vi "DestroyPublicEvents.vi"(8 "error in (no error)":errorcluster, 11 "JKI.Robot.SMO":refnum<class "JKI.Robot.SMO.lvclass">) -> (0 "error out":errorcluster, 3 "JKI.Robot.SMO out":refnum<class "JKI.Robot.SMO.lvclass">)   [LabVIEW 2014, in "JKI.Robot.SMO.lvclass"]
doc: "JKI State Machine Objects (SMO) 1.0.0.5\nJKI - JKI\nCopyright (c) 2016, JKI"
uses:
  JKI.Robot.SMO.lvclass
  JKI.Robot.SMO.Base/JKI.Robot.SMO.Base.lvclass
panel:
  # "For instructions on how to use the JKI State Machine Objects, examples and video tutorials, visit:\nhttp://jki.net/state-machine-objects/\n\nJKI State Machine Objects™\nhttp://jki.net/state-machine-objects/\nCopyright (C) 2005-2015, JKI <info@jki.net>\nALL RIGHTS RESERVED"
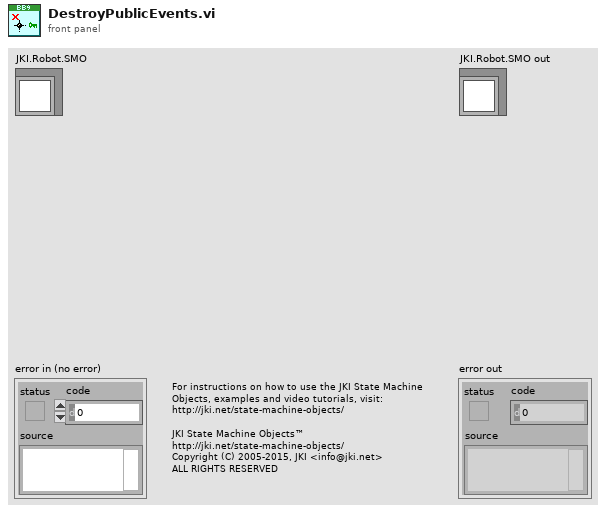
[diagram p1: front panel]
types:
  T1 = typedef "JKI.Robot.SMO.lvclass/PublicEvents--Cluster.ctl" = cluster{"Data Changed":refnum<user-event>}
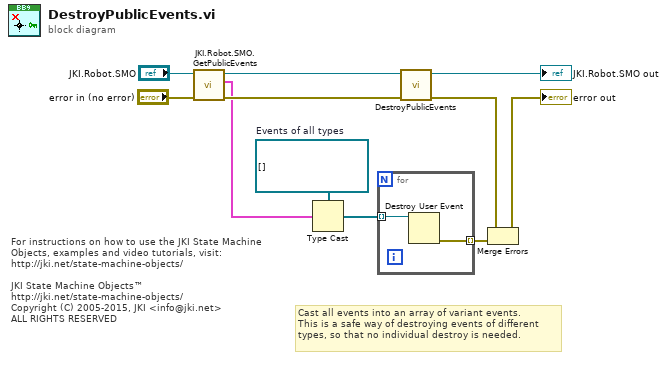
[diagram p0: block diagram]
diagram:
  w3 = refnum<user-event>[] []  # Events of all types
  # "For instructions on how to use the JKI State Machine Objects, examples and video tutorials, visit:\nhttp://jki.net/state-machine-objects/\n\nJKI State Machine Objects™\nhttp://jki.net/state-machine-objects/\nCopyright (C) 2005-2015, JKI <info@jki.net>\nALL RIGHTS RESERVED"
  # "Cast all events into an array of variant events.\nThis is a safe way of destroying events of different\ntypes, so that no individual destroy is needed."
  n1 = call "JKI.Robot.SMO.GetPublicEvents.vi"("error in (no error)"="error in (no error)", "JKI.Robot.SMO"="JKI.Robot.SMO") -> ("error out"=w7:errorcluster, "SMO.ByRefWithEvents Public Events"=w1:T1, "JKI.Robot.SMO out"=w9:refnum<class "JKI.Robot.SMO.lvclass">)  [unwired: 7 in]
  n2 = Type Cast(type=w3, x=w1) -> (*(type *) &x=w4:refnum<user-event>[])
  n3 = for {
    tunnel: w4 -> [w13] mode=indexing
    tunnel: [w12] -> w2 mode=indexing
    n4 = Destroy User Event(user event=w13) -> (error out=w12:errorcluster)  [unwired: 1 in]
  }
  n5 = call-parent "DestroyPublicEvents.vi"("error in (no error)"=w7, "JKI.Robot.SMO.Base"=w9) -> ("error out"=w6:errorcluster, "JKI.Robot.SMO.Base out"=→"JKI.Robot.SMO out":refnum<class "JKI.Robot.SMO.lvclass">)  [unwired: 8 in]
  n6 = Merge Errors(w6, w2) -> (→"error out":errorcluster)
